vi "2 LED Serial Sequence.vi"(8 "Tag Name 2":string="Boolean processing result 0", 9 "Tag Name 1":string="Boolean processing result 0", 10 "Name":string="Led Sequence") -> (2 "Sequence out":refnum<class "Sequence Config.lvclass">)   [LabVIEW 2015, in "Sequencer Module tests.lvlib"]
uses:
  Sequencer Module tests.lvlib
  classes/Sequence/Config/Sequence Config.lvclass
  <vilib>/NI/Tag Bus/tag/Data Type.ctl
  basic steps/Wait Step/Config/Wait Step Config.lvclass
  basic steps/Update Tag Step/Config/Update Tag Configuration/Update Tag Config.lvclass
  <vilib>/NI/Tag Bus Module Framework/channel/channel classification.ctl
  <vilib>/NI/Tag Bus/tag/tag descriptor.lvclass
  <vilib>/NI/Tag Bus Module Framework/channel/TBM channel.lvclass
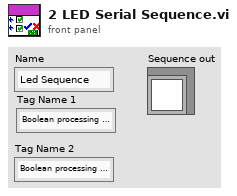
[diagram p1: front panel]
types:
  T1 = typedef "TBM channel.lvclass/channel classification.ctl" = enum16{"input data", "output data", "processing parameter", "processing result"}
  T2 = typedef "tag bus.lvlib/tag descriptor.lvclass/Data Type.ctl" = enum16{"Double", "Single", "I64", "I32", "I16", "I8", "U64", "U32", "U16", "U8", "Boolean", "String", "Array of Double", "Array of Single", "Array of I64", "Array of I32", "Array of I16", "Array of I8", "Array of U64", "Array of U32", "Array of U16", "Array of U8", "Array of Boolean", "Array of String"}
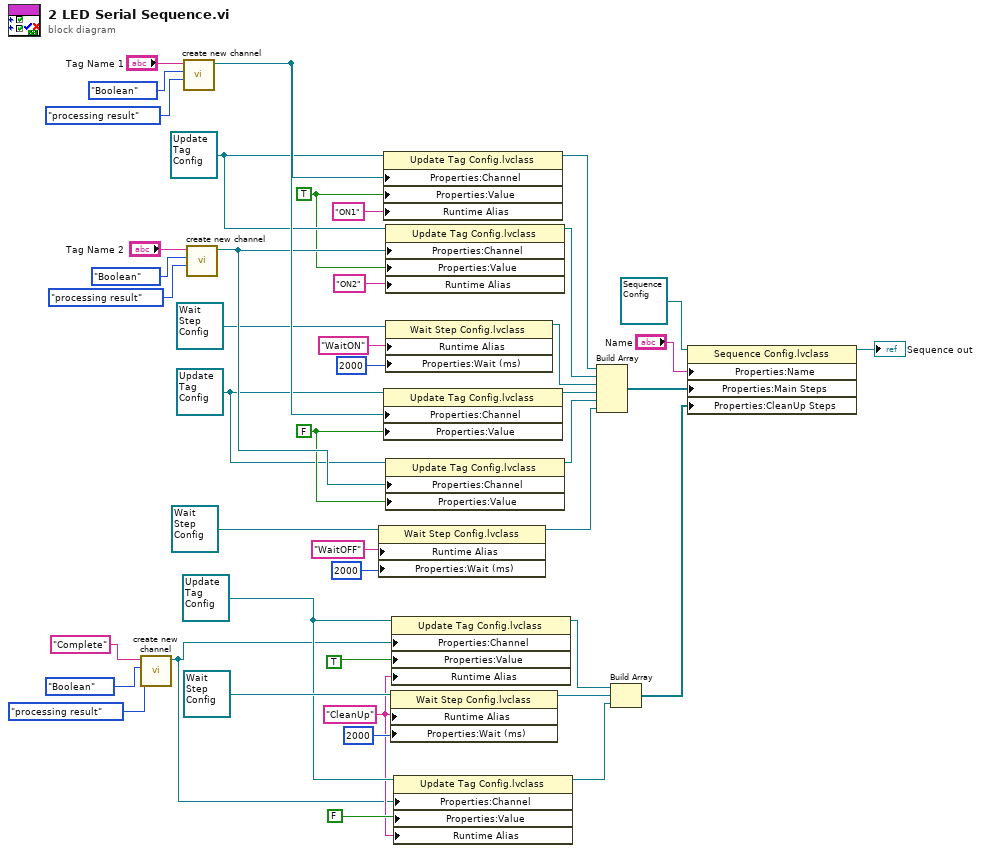
[diagram p0: block diagram]
diagram:
  w12 = refnum<class "Update Tag Config.lvclass"> refnum ("Update Tag Config.lvclass")
  w2 = "CleanUp" ("Runtime Alias")
  w18 = refnum<class "Update Tag Config.lvclass"> refnum ("Update Tag Config.lvclass")
  w29 = FALSE
  w30 = TRUE
  w31 = refnum<class "Update Tag Config.lvclass"> refnum ("Update Tag Config.lvclass")
  n1 = call <vilib>:"create new channel.vi"("channel classification"=channel_classification."processing result", "data type"=Data_Type."Boolean" ("Data Type"), "channel name"="Complete") -> ("channel"=w1:refnum<class "TBM channel.lvclass">)  [unwired: 8 in]
  n2 = call <vilib>:"create new channel.vi"("channel classification"=channel_classification."processing result", "data type"=Data_Type."Boolean" ("Data Type"), "channel name"="Tag Name 1") -> ("channel"=w36:refnum<class "TBM channel.lvclass">)  [unwired: 8 in]
  n3 = call <vilib>:"create new channel.vi"("channel classification"=channel_classification."processing result", "data type"=Data_Type."Boolean" ("Data Type"), "channel name"="Tag Name 2") -> ("channel"=w32:refnum<class "TBM channel.lvclass">)  [unwired: 8 in]
  n4 = property class="Wait Step Config.lvclass"(reference=refnum<class "Wait Step Config.lvclass"> refnum ("Wait Step Config.lvclass"), "Runtime Alias"="WaitOFF", "Properties:Wait (ms)"=u32 2000 ("Wait (ms)")) -> (reference out=w16:refnum<class "Wait Step Config.lvclass">)  [unwired: 1 in, 1 out]
  n5 = property class="Update Tag Config.lvclass"(reference=w31, "Properties:Channel"=w36, "Properties:Value"=w30, "Runtime Alias"="ON1") -> (reference out=w28:refnum<class "Update Tag Config.lvclass">)  [unwired: 1 in, 1 out]
  n6 = property class="Update Tag Config.lvclass"(reference=w18, "Properties:Channel"=w36, "Properties:Value"=w29) -> (reference out=w44:refnum<class "Update Tag Config.lvclass">)  [unwired: 1 in, 1 out]
  n7 = property class="Update Tag Config.lvclass"(reference=w31, "Properties:Channel"=w32, "Properties:Value"=w30, "Runtime Alias"="ON2") -> (reference out=w27:refnum<class "Update Tag Config.lvclass">)  [unwired: 1 in, 1 out]
  n8 = property class="Wait Step Config.lvclass"(reference=refnum<class "Wait Step Config.lvclass"> refnum ("Wait Step Config.lvclass"), "Runtime Alias"="WaitON", "Properties:Wait (ms)"=u32 2000 ("Wait (ms)")) -> (reference out=w15:refnum<class "Wait Step Config.lvclass">)  [unwired: 1 in, 1 out]
  n9 = property class="Update Tag Config.lvclass"(reference=w18, "Properties:Channel"=w32, "Properties:Value"=w29) -> (reference out=w26:refnum<class "Update Tag Config.lvclass">)  [unwired: 1 in, 1 out]
  n10 = property class="Wait Step Config.lvclass"(reference=refnum<class "Wait Step Config.lvclass"> refnum ("Wait Step Config.lvclass"), "Runtime Alias"=w2, "Properties:Wait (ms)"=u32 2000 ("Wait (ms)")) -> (reference out=w5:refnum<class "Wait Step Config.lvclass">)  [unwired: 1 in, 1 out]
  n11 = property class="Update Tag Config.lvclass"(reference=w12, "Properties:Channel"=w1, "Properties:Value"=TRUE, "Runtime Alias"=w2) -> (reference out=w6:refnum<class "Update Tag Config.lvclass">)  [unwired: 1 in, 1 out]
  n12 = property class="Update Tag Config.lvclass"(reference=w12, "Properties:Channel"=w1, "Properties:Value"=FALSE, "Runtime Alias"=w2) -> (reference out=w4:refnum<class "Update Tag Config.lvclass">)  [unwired: 1 in, 1 out]
  n13 = Build Array(w28, w27, w15, w44, w26, w16) -> (w43:refnum<class "Step Config.lvclass">[])
  n14 = Build Array(w6, w5, w4) -> (w3:refnum<class "Step Config.lvclass">[])
  n15 = property class="Sequence Config.lvclass"(reference=refnum<class "Sequence Config.lvclass"> refnum ("Sequence Config.lvclass"), "Properties:Name"="Name", "Properties:Main Steps"=w43, "Properties:CleanUp Steps "=w3) -> (reference out=→"Sequence out":refnum<class "Sequence Config.lvclass">)  [unwired: 1 in, 1 out]
